vi "drivetrain_ftsec_to_raw_real.vi"(11 "Drive Data":cluster{"Left":dbl, "Right":dbl}) -> (3 "Drive Data Out":cluster{"Left":dbl, "Right":dbl})   [LabVIEW 2011]
uses:
  drivetrain_globals.vi
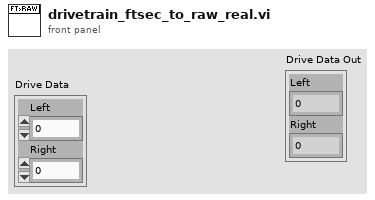
[diagram p1: front panel]
types:
  T1 = typedef "gear_shift_state.ctl" = enum16{"low", "high"}
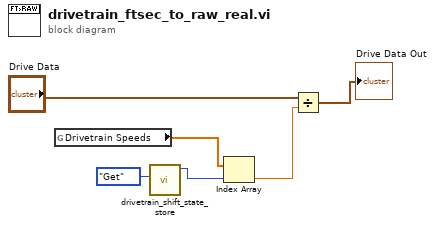
[diagram p0: block diagram]
diagram:
  n1 = global read "drivetrain_globals.vi" "Drivetrain Speeds"() -> (w5:dbl[])
  n2 = call "drivetrain_shift_state_store.vi"("data_store_mode"=enum16{"Set", "Get"}."Get") -> ("gear shift state out"=w4:T1)  [unwired: 10 in]
  n3 = Index Array(array=w5, index=w4) -> (element=w1:dbl)
  n4 = Divide(x="Drive Data", y=w1) -> (x/y=→"Drive Data Out":cluster{"Left":dbl, "Right":dbl})
